vi "Pockels-Power adjustment for AOL Z depth.vi"(9 "Laser power % corrected for depth":dbl[](array[numeric]), 11 "Z planes um (xi)":dbl[](array[numeric])=[90.0, 37.1, 7.0, 0.0, -68.2, -75.0, -113.0] format="%_6g") -> (1 "Laser power % corrected for AOL Z depth":dbl[](array[numeric]))   [LabVIEW 2017]
uses:
  Typedefs/Functional global standard states.ctl
  <vilib>/gmath/NI_Gmath.lvlib
panel:
  out "Cal data picked from this dwell time":dbl
  in  "Real AOL Z":string="-200\n-150\n-100\n-50\n0\n50\n100\n150\n180"
  in  "Efficiency % (Y)":string="66.20\t70.48\t57.81\t44.20\t34.27\t31.75\n73.24\t81.90\t71.88\t50.00\t48.95\t47.62\n84.51\t92.38\t87.50\t76.09\t67.13\t69.84\n90.14\t99.05\t98.44\t95.65\t90.91\t100.00\n95.77\t100.00\t100.00\t100.00\t100.00\t93.65\n100.00\t95.24\t92.19\t85.51\t78.32\t84.13\n95.77\t88.57\t76.56\t65.22\t55.94\t56.35\n90.14\t80.00\t62.50\t50.00\t41.96\t42.06\n88.73\t75.24\t55.47\t39.13\t36.36\t36.51"
  out "Efficiency % (yi)":dbl[](array[numeric]) format="%_6g"
  out "Real AOL Z (X)":dbl[](array[numeric]) format="%_6g"
  out "Efficiency % (Y)":dbl[](array[numeric]) format="%_6g"
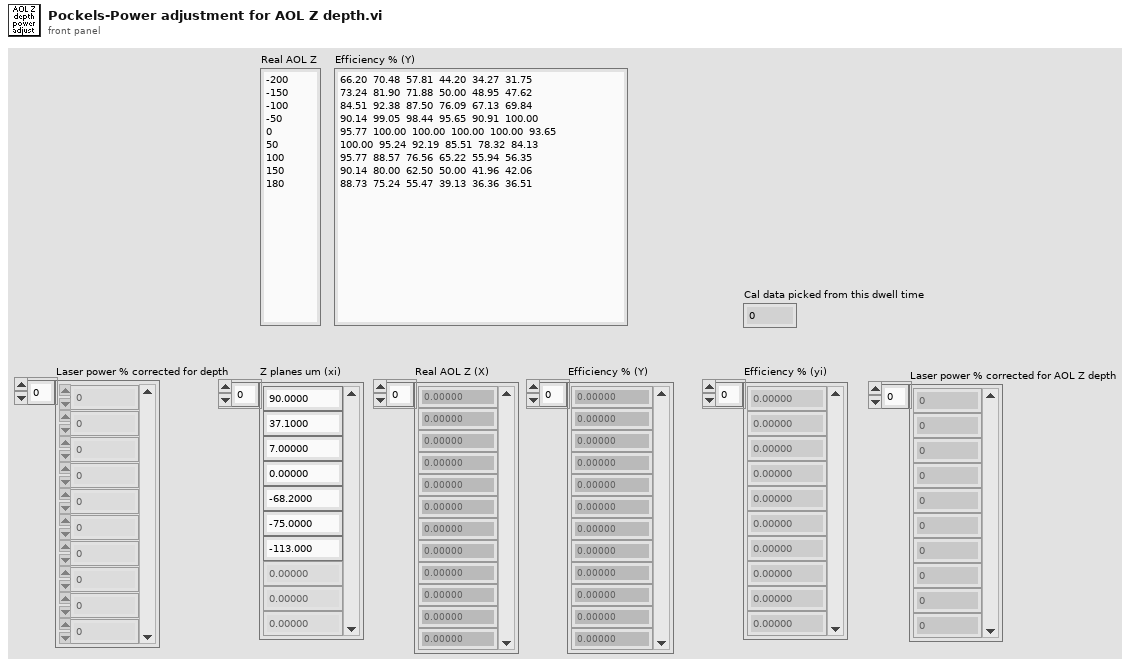
[diagram p1: front panel]
types:
  T1 = typedef "Functional global standard states.ctl" = enum16{"Initialise", "Read", "Write", "Load", "Save", "Clear"}
  T2 = typedef "AOL_Globals.ctl" = cluster{"Imaging Protocol":T3, "Number of POI":u16, "Number of Miniscans":u16, "Number of Trials":u16, "Number of Cycles ":u64, "# Averaged Frames":u16, "Laser power (%)":u8, "Pockels":dbl, "Acquisition Length (sec)":dbl, "Fill time (us)":dbl, "POI Dwell time (us)":dbl, "Miniscan Dwell time per pixel (us)":dbl, "PMT 1":dbl, "PMT 2":dbl, "Back Apperture":dbl, "Frame Size":T4, "Center Frequency":dbl, "Field of View":dbl, "DwellTime (us)":dbl, "Wavelength (nm)":dbl, "Zoom":dbl, "AOL Z":dbl, "AOL Mode":T5, "GridXY":dbl, "GridZ":dbl, "TriggerPeriod (sec)":dbl, "Number of Pixels in Miniscan":u16, "Experiment folder path":path, "X centre":dbl, "Y centre":dbl, "Angle (degrees)":dbl, "Plane Mode":T6, "Threshold":u16[], "Regenerate Chirps":bool, "Rectangle ROI length (pixels)":u16, "Rectangle ROI height (pixels)":u16, "AOD fill":u16, "StartupDelay":i32, "Samples Wait after Trigger":u16, "Slip Cycle":u32, "Add Cycle":bool}
  T3 = typedef "Imaging Protocols enum.ctl" = enum16{"AOL Z-Stack", "Motor Z Stack", "Functional Acquisition", "Single Plane Acquisition", "Volume Acquisition", "Live Imaging", "Live Plane Imaging", "Live Volume Imaging"}
  T4 = typedef "Frame Size.ctl" = u16
  T5 = typedef "AOL modes.ctl" = enum16{"Raster", "Structural", "Pointing", "Mini Scan", "Alignment"}
  T6 = typedef "Plane Mode.ctl" = u16
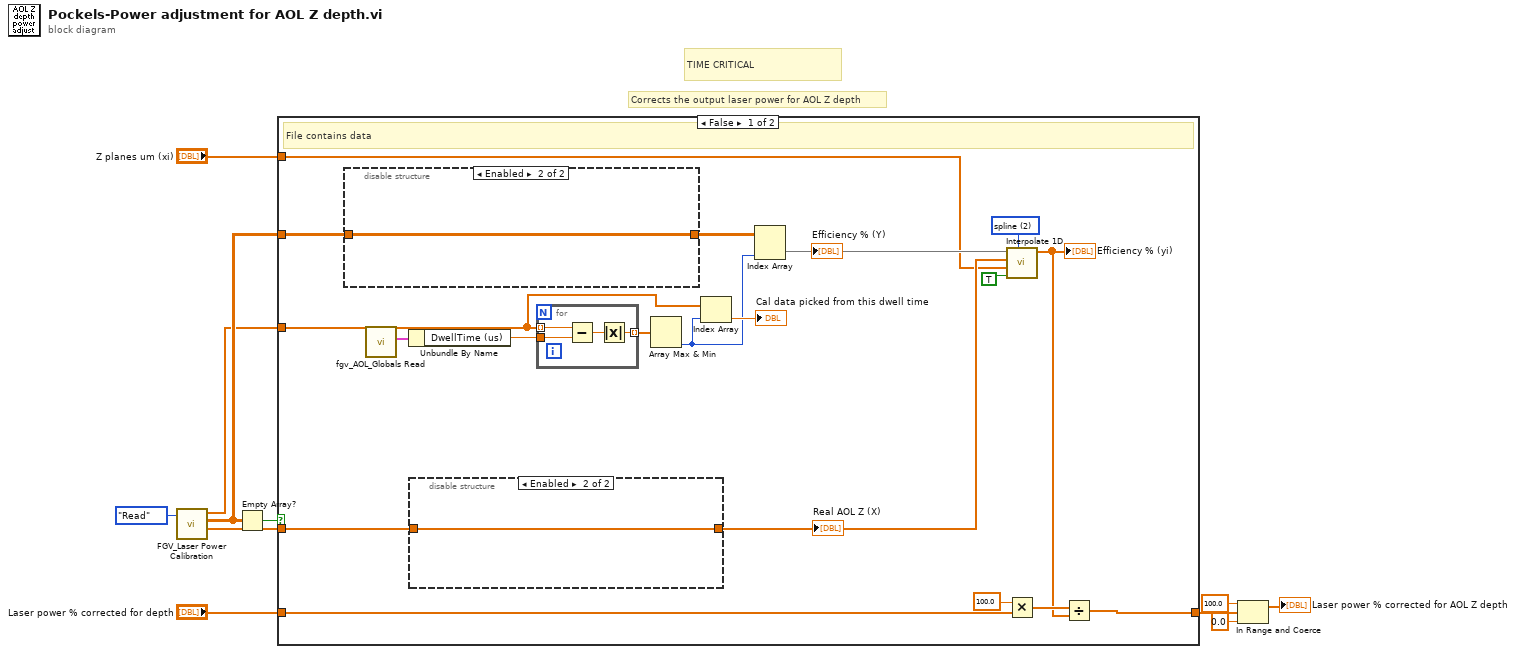
[diagram p0: block diagram]
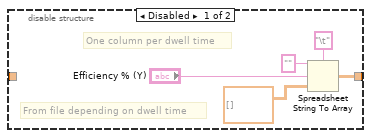
[diagram p2: hidden frame]
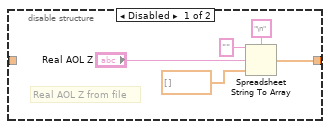
[diagram p3: hidden frame]
diagram:
  # "TIME CRITICAL"
  # "Corrects the output laser power for AOL Z depth"
  n1 = call "FGV_Laser Power Calibration.vi"("Function"=Functional_global_standard_states."Read") -> ("Real AOL Z"=w9:dbl[], "Calibration Data (% efficiency)"=w8:dbl[][], "Dwell time values (us)"=w6:dbl[])  [unwired: 7 in, 1 out]
  n2 = Empty Array?(array=w8) -> (empty?=w7:bool)
  n3 = case shown="False" w7 {
    tunnel: "Laser power % corrected for depth" -> [w23 w47]
    tunnel: [w12 w47] -> w2
    tunnel: w9 -> [w20 _]
    tunnel: w8 -> [w19 _]
    tunnel: w6 -> [w16 _]
    tunnel: "Z planes um (xi)" -> [w13 _]
    frame False {
      w26 = 2 items=["nearest", "linear", "spline", "cubic Hermite", "Lagrange"] ("method")
      # "File contains data"
      n4 = disable-structure shown="Enabled" {
        disable-tunnel: [w36 w40] -> w29
        disable-tunnel: w19 -> [_ w40]
        frame Disabled {
          # "One column per dwell time"
          # "From file depending on dwell time"
          n5 = Spreadsheet String To Array(delimiter (Tab)="\t", format string="", spreadsheet string="Efficiency % (Y)", array type (2D Dbl)=dbl[][] [] ("Efficiency % (Y)")) -> (array=w36:dbl[][])
        }
        frame Enabled {
        }
      }
      n6 = call "fgv_AOL_Globals Read.vi"() -> ("AOL_Globals"=w30:T2)  [unwired: 9 in, 2 out]
      n7 = Unbundle By Name(w30) -> ("DwellTime (us)"=w18:dbl)
      n8 = disable-structure shown="Enabled" {
        disable-tunnel: [w42 w46] -> w27
        disable-tunnel: w20 -> [_ w46]
        frame Disabled {
          # "Real AOL Z from file"
          n9 = Spreadsheet String To Array(delimiter (Tab)="\n", format string="", spreadsheet string="Real AOL Z", array type (2D Dbl)=dbl[] [] ("Efficiency % (Y)")) -> (array=w42:dbl[])
        }
        frame Enabled {
        }
      }
      "Real AOL Z (X)" <- w27
      n10 = for {
        tunnel: w16 -> [w34] mode=indexing
        tunnel: w18 -> [w33]
        tunnel: [w31] -> w17 mode=indexing
        n11 = Subtract(x=w34, y=w33) -> (x-y=w32:dbl)
        n12 = Absolute Value(x=w32) -> (abs(x)=w31:dbl)
      }
      n13 = Array Max & Min(array=w17) -> (min index (indices)=w14:i32)  [unwired: 3 out]
      n14 = Index Array(array=w16, index=w14) -> (element=→"Cal data picked from this dwell time":dbl)
      n15 = Index Array(array=w29, index (col)=w14) -> (element=w28:dbl[])  [unwired: 1 in]
      "Efficiency % (Y)" <- w28
      n16 = call <vilib>:"Interpolate 1D.vi"("method"=w26, "X is monotonic"=TRUE, "xi"=w13, "X"=w27, "Y"=w28) -> ("yi"=w21:dbl[])  [unwired: 4 in, 2 out]
      "Efficiency % (yi)" <- w21
      n17 = Multiply(x=100.0, y=w23) -> (x*y=w24:dbl[])
      n18 = Divide(x=w24, y=w21) -> (x/y=w12:dbl[])
    }
    frame True {
      # "File is empty"
    }
  }
  n19 = In Range and Coerce(upper limit=100.0, x=w2, lower limit=0.0) -> (coerced(x)=→"Laser power % corrected for AOL Z depth":dbl[])  [unwired: 1 out]
